vi "connect_to _device.vi"() -> ()   [LabVIEW 2012]
uses:
  hidapi_32bits.dll
panel:
  out "connectToDeviceByIndex":u16
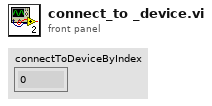
[diagram p1: front panel]
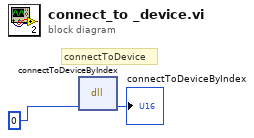
[diagram p0: block diagram]
diagram:
  # "connectToDevice"
  n1 = dll-call lib="C:/All_Data/mikrocont/Project1/New_controller__Jan_2015/LabView_Aug_2015/hidapi_32bits.dll" fn="connectToDeviceByIndex"("connectToDeviceByIndex"=u16 0 ("vendorId")) -> ("connectToDeviceByIndex"=→"connectToDeviceByIndex":u16)  [unwired: 4 in, 2 out]
